vi "Destroy Request Events.vi"(8 "error in":errorcluster) -> (0 "error out":errorcluster)   [LabVIEW 2025, in "Scripting Server.lvlib"]
doc: "Destroy the requests user events, even if there is an incoming error.\n\n<b>NOTE</b>: The contents of this VI are automatically generated and modified by the <b>Tools > DQMH Consortium > DQMH</b> utilities. Consider using those utilities instead of making your own modifications to this VI.\n_____\nBased on DQMH Dev Tools: Project Template 7.1.0.1503."
uses:
  Scripting Server.lvlib
panel:
  # "NOTE: The contents of this VI are automatically generated and modified by the Tools > DQMH Consortium > DQMH utilities. Consider using those utilities instead of making your own modifications to this VI."
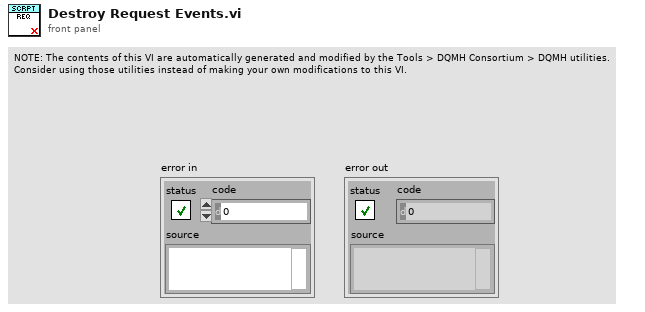
[diagram p1: front panel]
types:
  T1 = typedef "Scripting Server.lvlib/Request Events--cluster.ctl" = cluster{"Stop Module":refnum<user-event>, "Show Panel":refnum<user-event>, "Hide Panel":refnum<user-event>, "Get Module Execution Status":refnum<user-event>, "Show Diagram":refnum<user-event>, "New VI":refnum<user-event>, "Add Object":refnum<user-event>, "Connect Objects":refnum<user-event>, "Get Object Terminals":refnum<user-event>, "get vi error list":refnum<user-event>, "Cleanup VI":refnum<user-event>, "create_control":refnum<user-event>, "Run VI":refnum<user-event>, "add_to_selection":refnum<user-event>, "clear_selection_list":refnum<user-event>, "remove_from_selection":refnum<user-event>, "enclose_selection":refnum<user-event>, "rename_object":refnum<user-event>, "set_value":refnum<user-event>, "delete_object":refnum<user-event>, "save_vi":refnum<user-event>, "get_structure_diagram":refnum<user-event>, "add_subvi":refnum<user-event>, "connect_to_pane":refnum<user-event>, "get_object_help":refnum<user-event>, "get_loop_conditional_terminal":refnum<user-event>, "show_conditional_terminal":refnum<user-event>, "get_loop_iteration_terminal":refnum<user-event>, "Read Config Data":refnum<user-event>, "get_allowed_paths":refnum<user-event>, "create_project":refnum<user-event>, "Set Allowed Paths":refnum<user-event>}
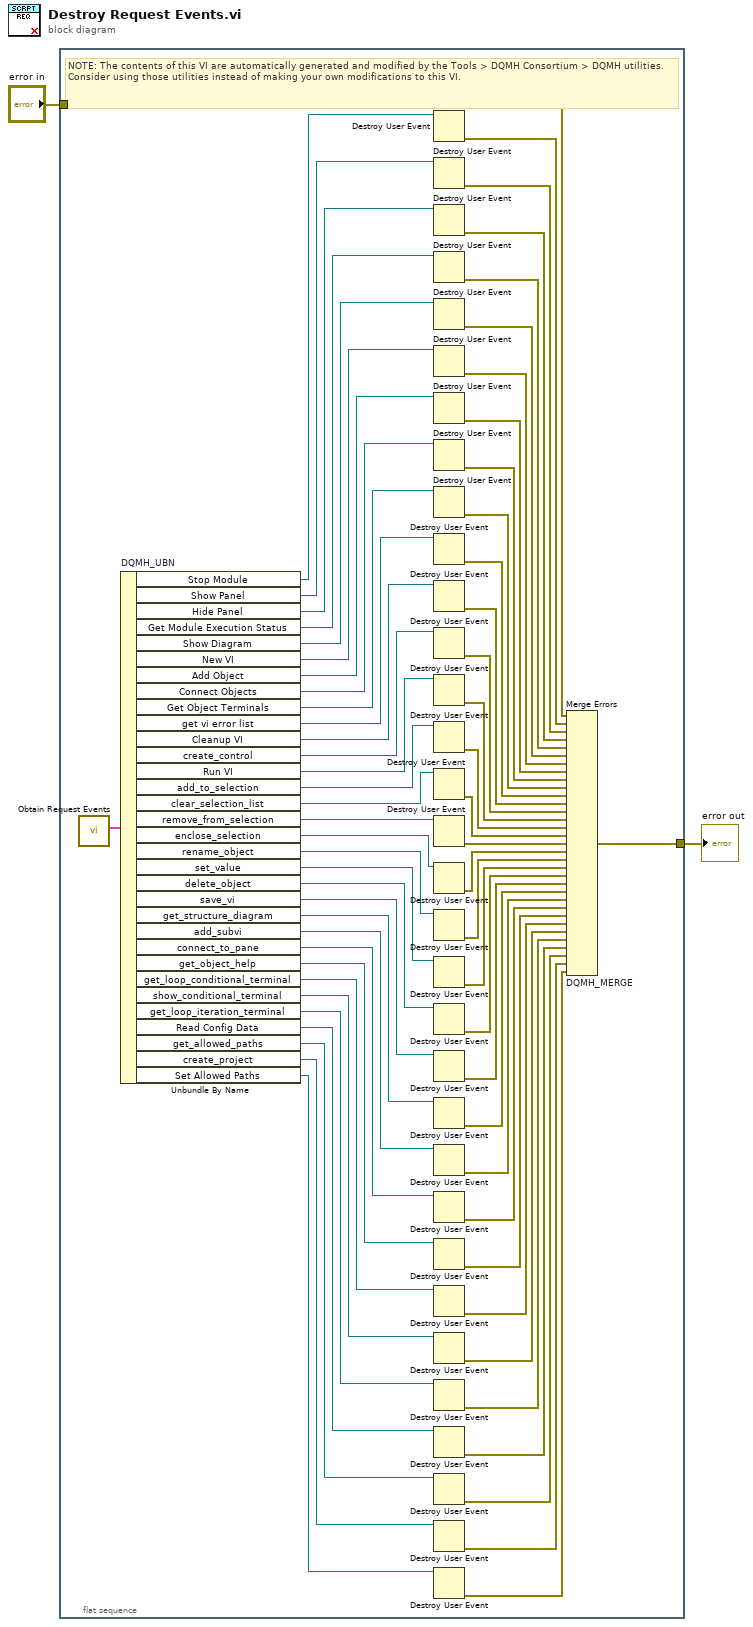
[diagram p0: block diagram]
diagram:
  n1 = flat-sequence {
    tunnel: [w68] -> w2
    tunnel: "error in" -> [w61]
    frame #0 {
      # "NOTE: The contents of this VI are automatically generated and modified by the Tools > DQMH Consortium > DQMH utilities. Consider using those utilities instead of making your own modifications to this VI."
      n2 = call "Obtain Request Events.vi"() -> ("Scripting Server Request Events"=w67:T1)  [unwired: 10 in, 1 out]
      n3 = Unbundle By Name "DQMH_UBN"(w67) -> ("Stop Module"=w66:refnum<user-event>, "Show Panel"=w63:refnum<user-event>, "Hide Panel"=w62:refnum<user-event>, "Get Module Execution Status"=w59:refnum<user-event>, "Show Diagram"=w57:refnum<user-event>, "New VI"=w55:refnum<user-event>, "Add Object"=w53:refnum<user-event>, "Connect Objects"=w51:refnum<user-event>, "Get Object Terminals"=w49:refnum<user-event>, "get vi error list"=w47:refnum<user-event>, "Cleanup VI"=w45:refnum<user-event>, "create_control"=w43:refnum<user-event>, "Run VI"=w41:refnum<user-event>, "add_to_selection"=w39:refnum<user-event>, "clear_selection_list"=w37:refnum<user-event>, "remove_from_selection"=w35:refnum<user-event>, "enclose_selection"=w33:refnum<user-event>, "rename_object"=w31:refnum<user-event>, "set_value"=w29:refnum<user-event>, "delete_object"=w27:refnum<user-event>, "save_vi"=w25:refnum<user-event>, "get_structure_diagram"=w23:refnum<user-event>, "add_subvi"=w21:refnum<user-event>, "connect_to_pane"=w19:refnum<user-event>, "get_object_help"=w17:refnum<user-event>, "get_loop_conditional_terminal"=w15:refnum<user-event>, "show_conditional_terminal"=w13:refnum<user-event>, "get_loop_iteration_terminal"=w11:refnum<user-event>, "Read Config Data"=w9:refnum<user-event>, "get_allowed_paths"=w7:refnum<user-event>, "create_project"=w5:refnum<user-event>, "Set Allowed Paths"=w3:refnum<user-event>)
      n4 = Destroy User Event(user event=w66) -> (error out=w69:errorcluster)  [unwired: 1 in]
      n5 = Destroy User Event(user event=w63) -> (error out=w65:errorcluster)  [unwired: 1 in]
      n6 = Destroy User Event(user event=w62) -> (error out=w64:errorcluster)  [unwired: 1 in]
      n7 = Destroy User Event(user event=w59) -> (error out=w60:errorcluster)  [unwired: 1 in]
      n8 = Destroy User Event(user event=w57) -> (error out=w58:errorcluster)  [unwired: 1 in]
      n9 = Destroy User Event(user event=w55) -> (error out=w56:errorcluster)  [unwired: 1 in]
      n10 = Destroy User Event(user event=w53) -> (error out=w54:errorcluster)  [unwired: 1 in]
      n11 = Destroy User Event(user event=w51) -> (error out=w52:errorcluster)  [unwired: 1 in]
      n12 = Destroy User Event(user event=w49) -> (error out=w50:errorcluster)  [unwired: 1 in]
      n13 = Destroy User Event(user event=w47) -> (error out=w48:errorcluster)  [unwired: 1 in]
      n14 = Destroy User Event(user event=w45) -> (error out=w46:errorcluster)  [unwired: 1 in]
      n15 = Destroy User Event(user event=w43) -> (error out=w44:errorcluster)  [unwired: 1 in]
      n16 = Destroy User Event(user event=w41) -> (error out=w42:errorcluster)  [unwired: 1 in]
      n17 = Destroy User Event(user event=w39) -> (error out=w40:errorcluster)  [unwired: 1 in]
      n18 = Destroy User Event(user event=w37) -> (error out=w38:errorcluster)  [unwired: 1 in]
      n19 = Destroy User Event(user event=w35) -> (error out=w36:errorcluster)  [unwired: 1 in]
      n20 = Destroy User Event(user event=w33) -> (error out=w34:errorcluster)  [unwired: 1 in]
      n21 = Destroy User Event(user event=w31) -> (error out=w32:errorcluster)  [unwired: 1 in]
      n22 = Destroy User Event(user event=w29) -> (error out=w30:errorcluster)  [unwired: 1 in]
      n23 = Destroy User Event(user event=w27) -> (error out=w28:errorcluster)  [unwired: 1 in]
      n24 = Destroy User Event(user event=w25) -> (error out=w26:errorcluster)  [unwired: 1 in]
      n25 = Destroy User Event(user event=w23) -> (error out=w24:errorcluster)  [unwired: 1 in]
      n26 = Destroy User Event(user event=w21) -> (error out=w22:errorcluster)  [unwired: 1 in]
      n27 = Destroy User Event(user event=w19) -> (error out=w20:errorcluster)  [unwired: 1 in]
      n28 = Destroy User Event(user event=w17) -> (error out=w18:errorcluster)  [unwired: 1 in]
      n29 = Destroy User Event(user event=w15) -> (error out=w16:errorcluster)  [unwired: 1 in]
      n30 = Destroy User Event(user event=w13) -> (error out=w14:errorcluster)  [unwired: 1 in]
      n31 = Destroy User Event(user event=w11) -> (error out=w12:errorcluster)  [unwired: 1 in]
      n32 = Destroy User Event(user event=w9) -> (error out=w10:errorcluster)  [unwired: 1 in]
      n33 = Destroy User Event(user event=w7) -> (error out=w8:errorcluster)  [unwired: 1 in]
      n34 = Destroy User Event(user event=w5) -> (error out=w6:errorcluster)  [unwired: 1 in]
      n35 = Destroy User Event(user event=w3) -> (error out=w4:errorcluster)  [unwired: 1 in]
      n36 = Merge Errors "DQMH_MERGE"(w61, w69, w65, w64, w60, w58, w56, w54, w52, w50, w48, w46, w44, w42, w40, w38, w36, w34, w32, w30, w28, w26, w24, w22, w20, w18, w16, w14, w12, w10, w8, w6, w4) -> (w68:errorcluster)
    }
  }
  "error out" <- w2
